vi "Consumer.vi"(8 "error in (no error)":errorcluster, 9 "Data":variant, 10 "Case ID":string, 11 "uService Template in":refnum<class "Kasli Server.lvclass">) -> (0 "error out":errorcluster, 3 "uService Template out":refnum<class "Kasli Server.lvclass">)   [LabVIEW 2020, in "TALOS.lvlib" / "Kasli Server.lvlib" / "Kasli Server.lvclass"]
uses:
  Kasli Server.lvclass
  Kasli Server Consumer Case Selector.ctl
  Ancestor/Ancestor/Ancestor.lvclass/Ancestor.ctl
  Support VIs/Generate Error.vi
  FGV/Error Memory/Get Error Description.vi
  Support VIs/Get PC name.vi
  Ancestor/Ancestor/Read ID.vi
  Support VIs/Get Class Name.vi
  <vilib>/Utility/error.llb/Clear Errors.vi
  FGV/Error Memory/Error Memory Core.vi
  <vilib>/AdvancedString/Delimited String to 1D String Array.vi
  Support VIs/Circus Root Path.vi
  FGV/Error Memory/Error Crt Lvl checker.vi
  FGV/Error Memory/Error Memory Core.vi/40c8088d-b597-4017-91af-faa98e00292e.vi
  FGV/Error Memory/Error Memory Core.vi/d4a3ab98-063c-4e44-b43d-fbdcfe6c2be2.vi
  Support VIs/Global Memory.vi
  <vilib>/Utility/LVClass/Get LV Class Name.vi
  Support VIs/Is in Packed Library.vi
  Support VIs/TALOS Root path.vi
  Support VIs/Read CSV worksheet.vi
  Support VIs/Global Constants.vi
  <vilib>/Utility/error.llb/General Error Handler.vi
  Support VIs/Error Log.vi
  Ancestor/Ancestor/Ancestor.lvclass
  <vilib>/Comparison/Equal/Equal Functor/Equal Functor.lvclass
  Father of all uServices/Father of all uServices/Father of all uServices.lvclass
  TALOS.lvlib
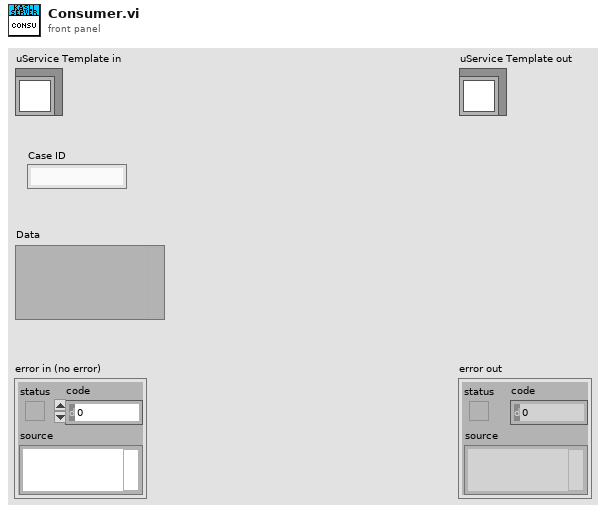
[diagram p1: front panel]
types:
  T1 = typedef "TALOS.lvlib/Kasli Server.lvlib/Kasli Server.lvclass/Kasli Server Consumer Case Selector.ctl" = enum16{"Send Message to Kasli"}
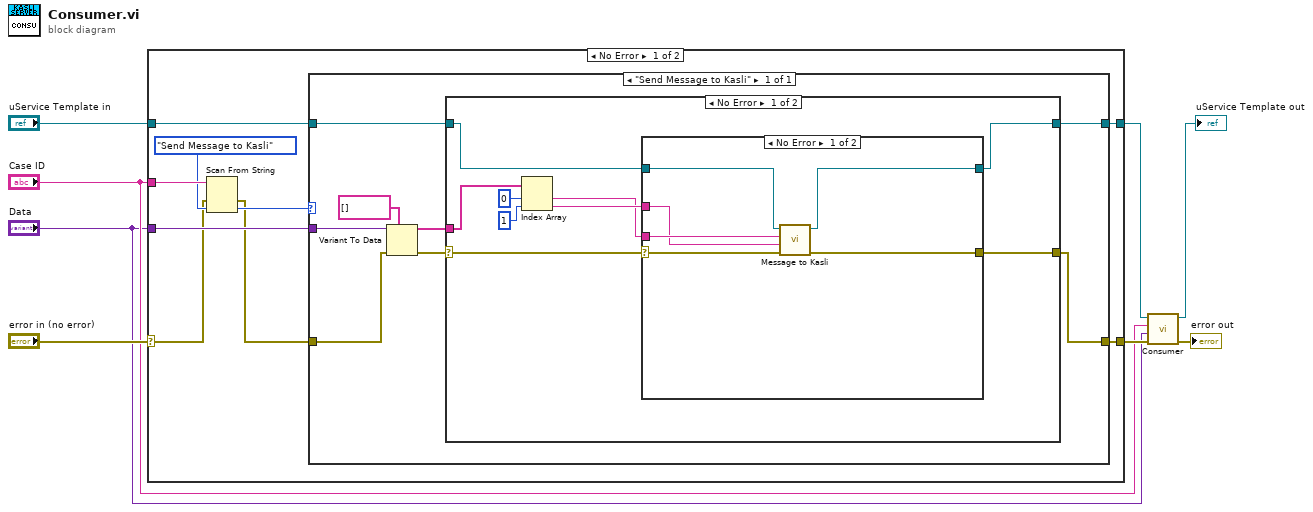
[diagram p0: block diagram]
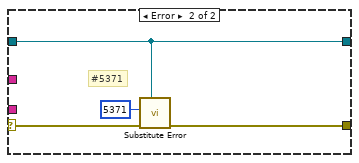
[diagram p2: hidden frame]
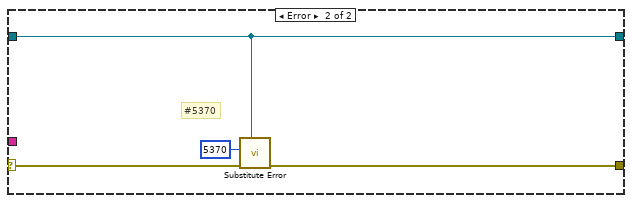
[diagram p3: hidden frame]
diagram:
  n1 = case shown="No Error" "error in (no error)" {
    selector: "error in (no error)" -> [w10 w49]
    tunnel: "uService Template in" -> [w16 w50]
    tunnel: [w14 w50] -> w4
    tunnel: [w15 w49] -> w3
    tunnel: "Case ID" -> [w13 _]
    tunnel: "Data" -> [w17 _]
    frame No Error {
      n2 = Scan From String(input string=w13, error in=w10, default 1=Kasli_Server_Consumer_Case_Selector."Send Message to Kasli") -> (error out=w9:errorcluster, output 1=w11:T1)  [unwired: 2 in, 2 out]
      n3 = case shown="\"Send Message to Kasli\"" w11 {
        tunnel: w17 -> [w25]
        tunnel: w9 -> [w23]
        tunnel: w16 -> [w21]
        tunnel: [w19] -> w15
        tunnel: [w20] -> w14
        frame "Send Message to Kasli" {
          n4 = Variant To Data(error in=w23, type=string[] [], Variant=w25) -> (data=w18:string[], error out=w22:errorcluster)
          n5 = case shown="No Error" w22 {
            selector: w22 -> [w31 w48]
            tunnel: w21 -> [w30 w47]
            tunnel: [w28 w47] -> w20
            tunnel: [w29 w45] -> w19
            tunnel: w18 -> [w34 _]
            frame No Error {
              n6 = Index Array(array=w34, index #1=0 ("index"), index #2=1 ("index")) -> (element #1=w26:string, element #2=w27:string)
              n7 = case shown="No Error" w31 {
                selector: w31 -> [w40 w44]
                tunnel: w30 -> [w36 w43]
                tunnel: [w37 w43] -> w28
                tunnel: [w35 w41] -> w29
                tunnel: w27 -> [w38 _]
                tunnel: w26 -> [w39 _]
                frame No Error {
                  n8 = call-dynamic "Message to Kasli.vi"("error in (no error)"=w40, "Message"=w38, "Kasli Name"=w39, "Father of all uServices in"=w36) -> ("error out"=w35:errorcluster, "Father of all uServices out"=w37:refnum<class "Kasli Server.lvclass">)  [unwired: 6 in]
                }
                frame Error {
                  # "#5371"
                  n9 = call "Substitute Error.vi"("LabVIEW Object"=w43, "error in (no error)"=w44, "Error Code"=5371) -> ("error out"=w41:errorcluster)  [unwired: 8 in]
                }
              }
            }
            frame Error {
              # "#5370"
              n10 = call "Substitute Error.vi"("LabVIEW Object"=w47, "error in (no error)"=w48, "Error Code"=5370) -> ("error out"=w45:errorcluster)  [unwired: 8 in]
            }
          }
        }
      }
    }
    frame Error {
    }
  }
  n11 = call-parent "Consumer.vi"("error in (no error)"=w3, "Data"="Data", "Case ID"="Case ID", "uService Template in"=w4) -> ("error out"=→"error out":errorcluster, "uService Template out"=→"uService Template out":refnum<class "Kasli Server.lvclass">)  [unwired: 6 in]
